vi "Write Current.vi"(8 "error in":errorcluster, 10 "Current":dbl, 11 "69X_79X in":refnum<class "69X_79X.lvclass">) -> (0 "error out":errorcluster, 3 "69X_79X out":refnum<class "69X_79X.lvclass">)   [LabVIEW 2019, in "69X_79X.lvlib" / "69X_79X.lvclass"]
uses:
  Library/69X_79X.lvclass
  C:/Users/Public/Documents/Development/builds/Instruments/PowerSupply.lvlibp/Library/PowerSupply.lvclass
  Library/69X_79X.lvclass/69X_79X.ctl
  Read Local Resource.vi
  builds/Instruments/PowerSupply.lvlibp/Library/PowerSupply.lvclass
  <instrlib>/Agilent N6900 N7900 Series/Agilent N6900 N7900 Series.lvlib
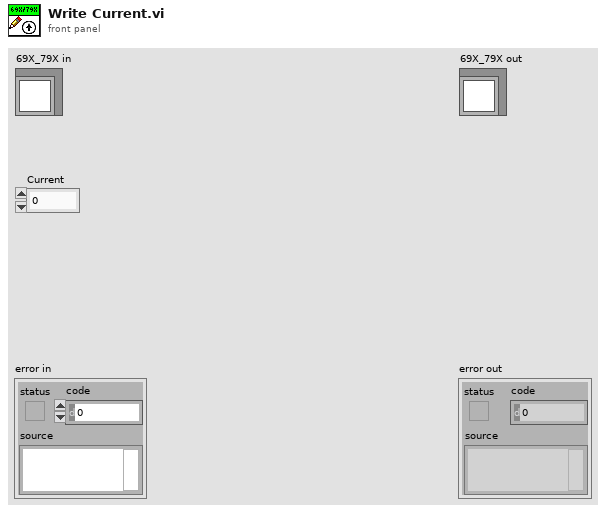
[diagram p1: front panel]
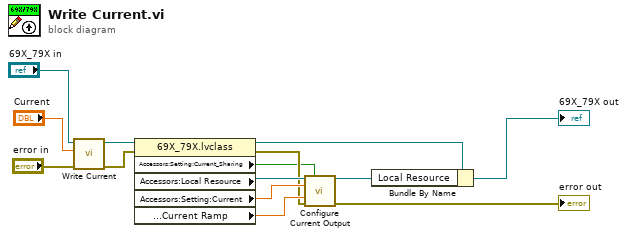
[diagram p0: block diagram]
diagram:
  n1 = call-parent "Write Current.vi"("error in"="error in", "Current"="Current", "PowerSupply in"="69X_79X in") -> ("error out"=w9:errorcluster, "PowerSupply out"=w11:refnum<class "69X_79X.lvclass">)  [unwired: 7 in]
  n2 = property class="69X_79X.lvclass"(reference=w11, error in=w9) -> (reference out=w10:refnum<class "69X_79X.lvclass">, error out=w2:errorcluster, "Accessors:Setting:Current_Sharing"=w1:bool, "Accessors:Local Resource"=w8:refnum<visa-resource-name>, "Accessors:Setting:Current"=w6:dbl, "Accessors:Setting:Ramp:Current Ramp"=w7:dbl)
  n3 = call <instrlib>:"Configure Current Output.vi"("VISA resource name"=w8, "Enable Parallel Unit Sharing (False)"=w1, "Current Immediate Amplitude (0 A)"=w6, "Current Slew (Inf)"=w7, "error in (no error)"=w2) -> ("VISA resource name out"=w3:refnum<visa-resource-name>, "error out"=→"error out":errorcluster)  [unwired: 9 in]
  n4 = Bundle By Name(cluster=w10, "Local Resource"=w3) -> (→"69X_79X out":refnum<class "69X_79X.lvclass">)
